vi "SIM900 Module Write.vi"(8 "Error In":errorcluster, 9 "Query":string, 10 "Slot":T1(ring), 11 "VISA Resource Name":refnum<visa-resource-name>="GPIB0::3::INSTR") -> (0 "Error Out":errorcluster {"code" format="%.0x"}, 3 "dup VISA Session":refnum<visa-resource-name>)   [LabVIEW 2020]
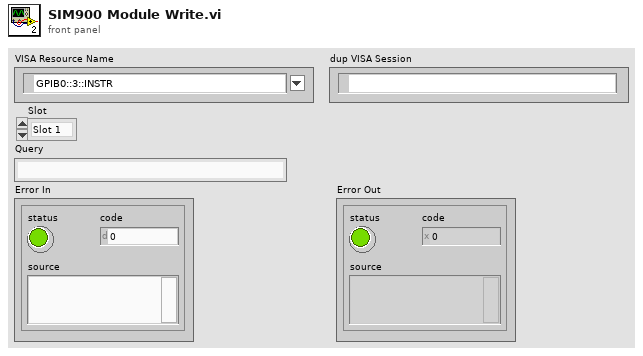
[diagram p1: front panel]
types:
  T1 = enum32{"Slot 1", "Slot 2", "Slot 3", "Slot 4", "Slot 5", "Slot 6", "Slot 7", "Slot 8"}
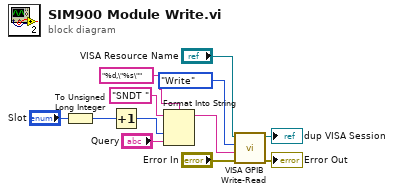
[diagram p0: block diagram]
diagram:
  n1 = To Unsigned Long Integer(number="Slot") -> (unsigned 32bit integer=w2:u32)
  n2 = Increment(x=w2) -> (x+1=w1:u32)
  n3 = Format Into String(format string="%d,\"%s\"", initial string="SNDT ", w1, "Query") -> (resulting string=w7:string)  [unwired: 1 in, 1 out]
  n4 = call "VISA GPIB Write-Read.vi"("error in (no error)"="Error In", "Command"=w7, "Action"=enum16{"Write", "Read", "Write & Read"}."Write", "VISA resource name"="VISA Resource Name") -> ("error out"=→"Error Out":errorcluster, "dup VISA Session"=→"dup VISA Session":refnum<visa-resource-name>)  [unwired: 4 in, 2 out]
